vi "ExConvertFile.vi"() -> ()   [LabVIEW 2010]
panel:
  in  "Output File Operation":u32=9
  in  "Output File Name":string
  in  "Output FileType":u32=67174400
  in  "stop":bool
  in  "Input File Operation":u32=6
  in  "Input File Name":string
  in  "Input FileType":u32=67371008
  out "error out":errorcluster
  in  "error in (no error)":errorcluster
  # "TIF   = 67174400\n  SPE = 67371008\n  PMI  = 67436544"
  # "NOTICE\n\nTHIS VI REQUIRES THAT THE TOOLKIT\nBE UNLOADED BY RUNNING THE\n VI EXCLOSEGLOBALCAM.VI\n BEFORE LEAVING LABVIEW."
  # "6 = Read Only"
  # "TIF   = 67174400\n  SPE = 67371008\n  PMI  = 67436544"
  # "9 = Open New / Write Only"
  # "ExConvertFile.vi\nThis VI will open the input file, display it and save\nit to the output file.  Note that the full path names\nmust be provided for both input and output files.\n\nThe STOP button must be used to end this VI.\nIt will correctly close the display window."
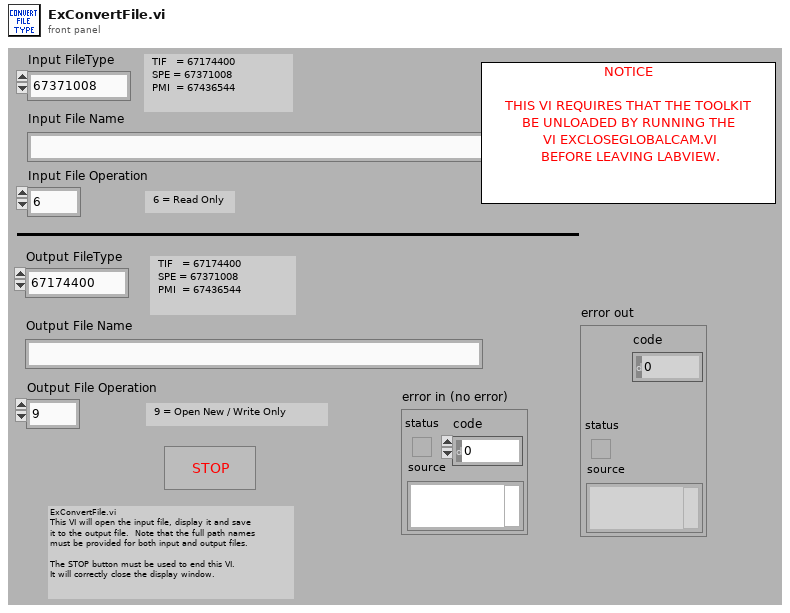
[diagram p1: front panel]
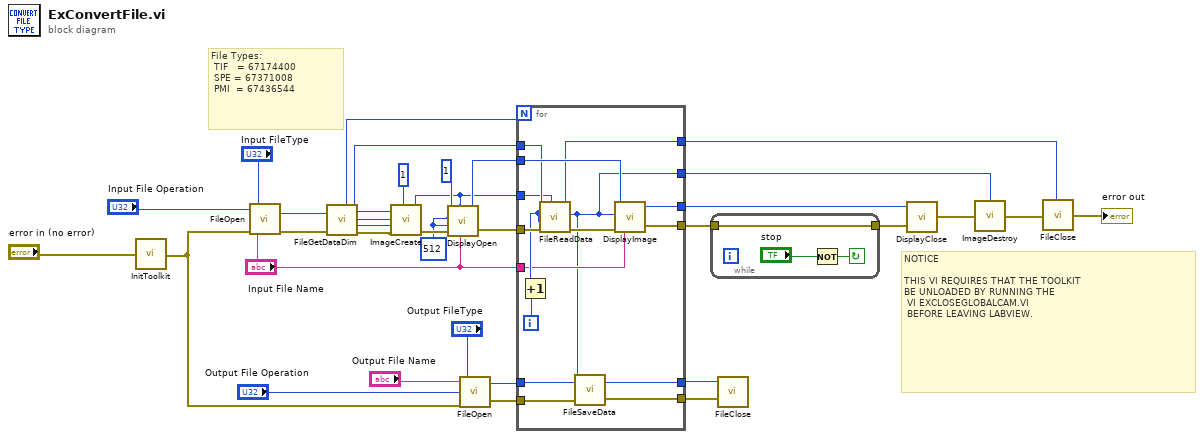
[diagram p0: block diagram]
diagram:
  w24 = 512
  # "NOTICE\n\nTHIS VI REQUIRES THAT THE TOOLKIT\nBE UNLOADED BY RUNNING THE\n VI EXCLOSEGLOBALCAM.VI\n BEFORE LEAVING LABVIEW."
  # "File Types:\n TIF   = 67174400\n SPE = 67371008\n PMI  = 67436544"
  n1 = call <userlib>:"InitToolkit.vi"("error in"="error in (no error)") -> ("error out"=w6:errorcluster)
  n2 = call <userlib>:"FileOpen.vi"("error in"=w6, "File Operations"="Input File Operation", "FileName"="Input File Name", "File Type"="Input FileType") -> ("error out"=w33:errorcluster, "File Handle"=w32:u32)
  n3 = call <userlib>:"FileGetDataDim.vi"("File Handle"=w32, "error in"=w33) -> ("Number of Frames"=w26:u32, "Data Type"=w28:u32, "File Handle"=w20:u32, "X dim"=w30:u32, "Y dim"=w29:u32, "error out"=w31:errorcluster)
  n4 = call <userlib>:"ImageCreate.vi"("X dimension"=w30, "Y dimension"=w29, "Data Type"=w28, "error in"=w31, "Number Of Frames"=1) -> ("Image Handle"=w19:u32, "error out"=w27:errorcluster)
  n5 = call <userlib>:"DisplayOpen.vi"("Display Title"="Input File Name", "Image Handle"=w19, "error in"=w27, "Display Height"=w24, "Display Width"=w24, "Display Type"=1) -> ("error out"=w22:errorcluster, "Display Handle"=w21:u32)
  n6 = call <userlib>:"FileOpen.vi"("error in"=w6, "File Operations"="Output File Operation", "FileName"="Output File Name", "File Type"="Output FileType") -> ("error out"=w4:errorcluster, "File Handle"=w5:u32)
  n7 = for {
    N: w26 -> [_]
    tunnel: w22 -> [w51]
    tunnel: w21 -> [w49]
    tunnel: w20 -> [w48]
    tunnel: w19 -> [w47]
    tunnel: [w41] -> w11
    tunnel: [w44] -> w18
    tunnel: [w43] -> w17
    tunnel: [w40] -> w14
    tunnel: "Input File Name" -> [w42]
    tunnel: w5 -> [w39]
    tunnel: [w38] -> w3
    tunnel: w4 -> [w37]
    tunnel: [w36] -> w2
    i -> [w46]
    n8 = Increment(x=w46) -> (x+1=w45:i32)
    n9 = call <userlib>:"FileReadData.vi"("File Handle"=w48, "Start Frame"=w45, "End Frame"=w45, "error in"=w51, "Image Handle"=w47) -> ("File Handle"=w43:u32, "Image Handle"=w40:u32, "error out"=w50:errorcluster)
    n10 = call <userlib>:"FileSaveData.vi"("error in"=w37, "Image Handle"=w40, "File Handle"=w39) -> ("error out"=w36:errorcluster, "File Handle"=w38:u32)
    n11 = call <userlib>:"DisplayImage.vi"("error in"=w50, "Title"=w42, "Image Handle"=w40, "Display Handle"=w49) -> ("error out"=w41:errorcluster, "Display Handle"=w44:u32)
  }
  n12 = while {
    tunnel: w11 -> [w54]
    tunnel: [w54] -> w12
    stop <- w52 continue-if-true
    n13 = Not(x="stop") -> (.not. x?=w52:bool)
  }
  n14 = call <userlib>:"FileClose.vi"("error in"=w2, "File Handle"=w3) -> ()  [unwired: 1 out]
  n15 = call <userlib>:"DisplayClose.vi"("error in"=w12, "Display Handle"=w18) -> ("error out"=w16:errorcluster)
  n16 = call <userlib>:"ImageDestroy.vi"("error in"=w16, "Data handle"=w14) -> ("error out"=w15:errorcluster)
  n17 = call <userlib>:"FileClose.vi"("error in"=w15, "File Handle"=w17) -> ("error out"=→"error out":errorcluster)
